vi "kvCanObjBufEnable.vi"(2 "error in (no error)":errorcluster, 3 "Object Handle":i32, 4 "Channel Handle (input only)":i32) -> (0 "error out":errorcluster, 1 "Channel Handle (output only)":i32)   [LabVIEW 2022 SP3]
doc: "Activates the object buffer so transmissions can start taking place based on the buffers configuration."
uses:
  canlib32.dll
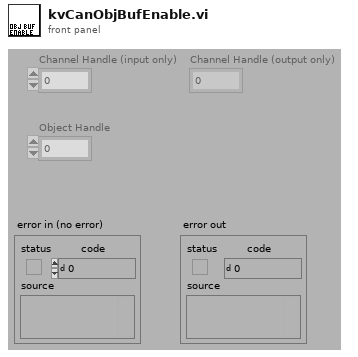
[diagram p1: front panel]
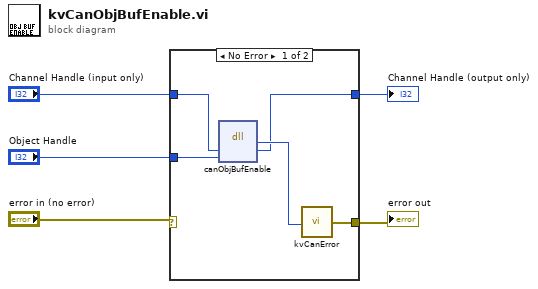
[diagram p0: block diagram]
diagram:
  n1 = case shown="No Error" "error in (no error)" {
    selector: "error in (no error)" -> [_ w11]
    tunnel: "Object Handle" -> [w8 _]
    tunnel: "Channel Handle (input only)" -> [w9 w12]
    tunnel: [w6 w12] -> w1
    tunnel: [w10 w11] -> w2
    frame No Error {
      n2 = dll-call lib="canlib32.dll" fn="canObjBufEnable"("channelHandle"=w9, "objectHandle"=w8) -> (w7:i32, "channelHandle"=w6:i32)  [unwired: 4 in, 2 out]
      n3 = call "kvCanError.vi"("error code"=w7) -> ("error out"=w10:errorcluster)
    }
    frame Error {
    }
  }
  "Channel Handle (output only)" <- w1
  "error out" <- w2
